vi "sub_USRP_MIMO_init_Rx.vi"(11 "Rx Parameters":T1={"IQ rate (Hz)"=200000.0, "Carrier frequency [Hz]"=1187500000.0, "Gain [dB]"=16.0, "Antenna"="RX1", "Rx device name"="192.168.10.4; 192.168.10.5;"} {"Gain [dB]" format="%#_6f"; "Carrier frequency [Hz]" format="%#_6p"; "IQ rate (Hz)" format="%#_6p"}) -> (0 "Error out":errorcluster, 3 "Rx Session handle out":refnum<k15>="192.168.10.3 (5)")   [LabVIEW 2012]
uses:
  <instrlib>/niUSRP/niUSRP Timestamp.ctl
  <instrlib>/niUSRP/niUSRP Configure Time Start Trigger.vi
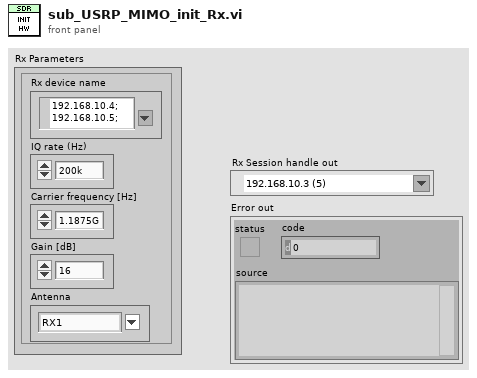
[diagram p1: front panel]
types:
  T1 = cluster{"IQ rate (Hz)":dbl, "Carrier frequency [Hz]":dbl, "Gain [dB]":dbl, "Antenna":string, "Rx device name":refnum<k15>}
  T2 = typedef "niUSRP Timestamp.ctl" = cluster{"whole seconds":u64, "fractional seconds":dbl}
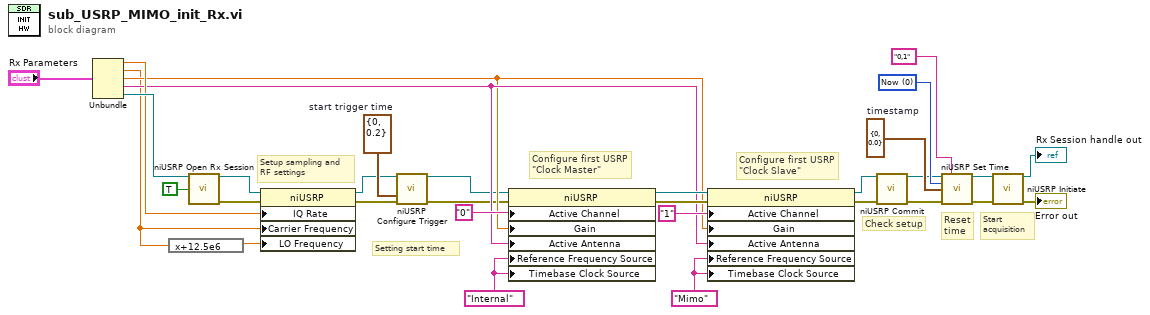
[diagram p0: block diagram]
diagram:
  w10 = T2 {"whole seconds"=0, "fractional seconds"=0.0}  # timestamp
  w9 = 0 items=["Now", "Next Timebase Edge"] ("apply timestamp")
  w30 = T2 {"whole seconds"=0, "fractional seconds"=0.2}  # start trigger time
  w22 = "Mimo" ("Clocking and Synchronization:Reference Frequency Source")
  w27 = "Internal" ("Clocking and Synchronization:Reference Frequency Source")
  # "Start\nacquisition"
  # "Reset\ntime"
  # "Check setup"
  # "Setting start time"
  # "Setup sampling and\nRF settings"
  # "Configure first USRP\n\"Clock Slave\""
  # "Configure first USRP\n\"Clock Master\""
  n1 = Unbundle("Rx Parameters") -> ("IQ rate (Hz)"=w29:dbl, "Carrier frequency [Hz]"=w1:dbl, "Gain [dB]"=w21:dbl, "Antenna"=w23:string, "Rx device name"=w31:refnum<k15>)
  n2 = expression code="x+12.5e6"(w1) -> (w2:dbl)
  n3 = call <instrlib>:"niUSRP Open Rx Session.vi"("device names"=w31, "reset"=TRUE) -> ("session handle out"=w20:refnum<k15>, "error out"=w19:errorcluster)  [unwired: 12 in]
  n4 = property class="niUSRP"(reference=w20, error in=w19, "IQ Rate"=w29, "Carrier Frequency"=w1, "LO Frequency"=w2) -> (reference out=w18:refnum<k15>, error out=w17:errorcluster)
  n5 = call-poly <instrlib>:"niUSRP Configure Trigger.vi"("session handle"=w18, "start trigger time"=w30, "error in (no error)"=w17) -> ("session handle out"=w16:refnum<k15>, "error out"=w15:errorcluster)  [unwired: 11 in]
  n6 = property class="niUSRP"(reference=w16, error in=w15, "Active Channel"="0", "Gain"=w21, "Active Antenna"=w23, "Reference Frequency Source"=w27, "Timebase Clock Source"=w27) -> (reference out=w25:refnum<k15>, error out=w24:errorcluster)
  n7 = property class="niUSRP"(reference=w25, error in=w24, "Active Channel"="1", "Gain"=w21, "Active Antenna"=w23, "Reference Frequency Source"=w22, "Timebase Clock Source"=w22) -> (reference out=w14:refnum<k15>, error out=w13:errorcluster)
  n8 = call <instrlib>:"niUSRP Commit.vi"("session handle"=w14, "error in (no error)"=w13) -> ("session handle out"=w6:refnum<k15>, "error out"=w5:errorcluster)  [unwired: 12 in]
  n9 = call <instrlib>:"niUSRP Set Time.vi"("session handle"=w6, "channel list"="0,1", "apply timestamp"=w9, "timestamp"=w10, "error in (no error)"=w5) -> ("session handle out"=w12:refnum<k15>, "error out"=w11:errorcluster)  [unwired: 9 in]
  n10 = call <instrlib>:"niUSRP Initiate.vi"("session handle"=w12, "error in (no error)"=w11) -> ("session handle out"=→"Rx Session handle out":refnum<k15>, "error out"=→"Error out":errorcluster)  [unwired: 12 in]
